vi "Read Digital Voltmeter.vi"(8 "error in (no error)":errorcluster, 11 "VISA resource name":refnum<visa-resource-name>) -> (0 "error out":errorcluster, 1 "5-digit Frequency":dbl, 2 "3-digit DVM":dbl, 3 "VISA resource name out":refnum<visa-resource-name>)   [LabVIEW 2015, in "Agilent 2000 3000 X-Series.lvlib"]
doc: "Returns the displayed value of the digital voltmeter (DVM)."
uses:
  <instrlib>/Agilent 2000 3000 X-Series/Agilent 2000 3000 X-Series.lvlib
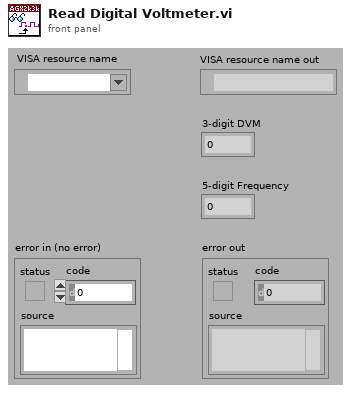
[diagram p1: front panel]
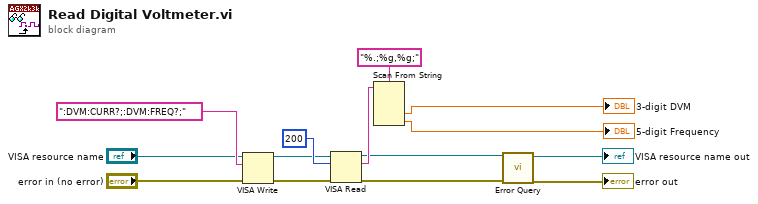
[diagram p0: block diagram]
diagram:
  n1 = VISA Write(VISA resource name="VISA resource name", write buffer=":DVM:CURR?;:DVM:FREQ?;", error in (no error)="error in (no error)") -> (VISA resource name out=w6:refnum<visa-resource-name>, error out=w5:errorcluster)  [unwired: 1 out]
  n2 = VISA Read(VISA resource name=w6, byte count=u32 200, error in (no error)=w5) -> (VISA resource name out=w2:refnum<visa-resource-name>, read buffer=w8:string, error out=w1:errorcluster)  [unwired: 1 out]
  n3 = Scan From String(format string="%.;%g,%g;", input string=w8) -> (output 1=→"3-digit DVM":dbl, output 2=→"5-digit Frequency":dbl)  [unwired: 2 in, 5 out]
  n4 = call <instrlib>:"Error Query.vi"("error in (no error)"=w1, "VISA resource name"=w2) -> ("error out"=→"error out":errorcluster, "VISA resource name out"=→"VISA resource name out":refnum<visa-resource-name>)  [unwired: 8 out]
